vi "fgv.vi"(10 "Motor Speed In":dbl, 11 "Mode":enum16{"Initialize", "Set", "Read"}(ring)) -> (3 "Motor Speed Out":dbl)   [LabVIEW 2014]
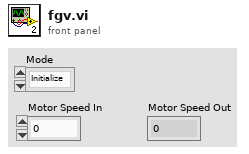
[diagram p1: front panel]
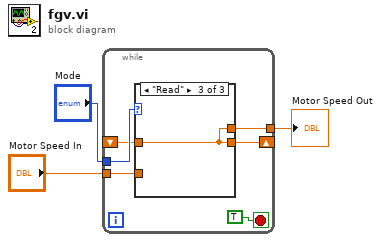
[diagram p0: block diagram]
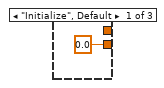
[diagram p2: hidden frame]
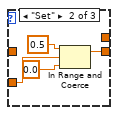
[diagram p3: hidden frame]
diagram:
  n1 = while {
    shift-right: [w7] -> _
    shift-left: _ -> [w5]
    tunnel: "Mode" -> [w8]
    tunnel: "Motor Speed In" -> [w6]
    tunnel: [w4] -> w1
    stop <- TRUE stop-if-true
    n2 = case shown="\"Read\"" w8 {
      tunnel: [0.0 w11 w15] -> w7
      tunnel: w6 -> [_ w14 _]
      tunnel: w5 -> [_ _ w15]
      tunnel: [_ _ w15] -> w4
      frame "Initialize", Default {
      }
      frame "Set" {
        n3 = In Range and Coerce(upper limit=0.5, x=w14, lower limit=0.0) -> (coerced(x)=w11:dbl)  [unwired: 1 out]
      }
      frame "Read" {
      }
    }
  }
  "Motor Speed Out" <- w1
